vi "Tell Child.vi"(4 "Priority":bool, 6 "UID":string, 7 "Actor in":refnum<class "Actor.lvclass">) -> (0 "Error out":errorcluster)   [LabVIEW 2025, in "_Template.lvlib" / "Templates.lvlib" / "TEMPLATE Msg.lvlib"]
uses:
  TEMPLATE Msg.lvlib
  jettl/jettl/Actor/Actor.lvclass
  TEMPLATE Msg/TEMPLATE Msg.lvclass
  C:/git/jettl/src/jettl Tools/_Template/Templates/TEMPLATE Msg/TEMPLATE Msg/TEMPLATE Msg.lvclass
  C:/git/jettl/src/jettl/jettl/Msg/Msg.lvclass
  jettl/jettl/jettl.lvlib
panel:
  # "This front panel should not be manipulated."
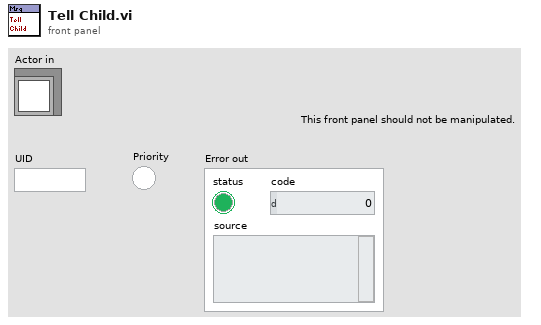
[diagram p1: front panel]
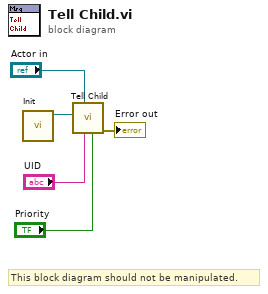
[diagram p0: block diagram]
diagram:
  # "This block diagram should not be manipulated."
  n1 = call "Init.vi"() -> ("TEMPLATE Msg out"=w4:refnum<class "TEMPLATE Msg.lvclass">)  [unwired: 11 in]
  n2 = call "Tell Child.vi"("Priority"="Priority", "UID"="UID", "Actor in"="Actor in", "Msg"=w4) -> ("Error out"=→"Error out":errorcluster)  [unwired: 7 in]
